vi "glavni_program.vi"() -> ()   [LabVIEW 2019]
uses:
  vrste_kafe.ctl
  stanja.ctl
  <vilib>/DAQmx/read.llb/DAQmx Read (Analog 1D DBL 1Chan NSamp).vi
  <vilib>/DAQmx/read.llb/DAQmx Read (Analog DBL 1Chan 1Samp).vi
  <vilib>/DAQmx/miscellaneous.llb/DAQmx Fill In Error Info.vi
  <vilib>/DAQmx/create/channels.llb/DAQmx Create Channel (AI-Voltage-Basic).vi
  <vilib>/DAQmx/configure/timing.llb/DAQmx Timing (Sample Clock).vi
panel:
  out "temperatura":dbl
  out "zapremina":dbl
  out "vreme kafe":i32
  in  "izbor kraci/duzi":bool
  in  "duzi espresso":bool
  out "vreme zagrevanja[ms]":u32
  out "start time":u32
  in  "stop":bool
  in  "Broj kafa":T1
  in  "Izbor kafe":T2
  in  "Ukljuci":bool
  out "L2":bool
  in  "Otkloni gresku":bool
  in  "Pravi kafu":bool
  in  "Zagrej vodu":bool
  in  "Ubaci kapsulu":bool
  out "Lampice":T3
  in  "Dopuni":bool
  out "L1":bool
  # "kraći espresso"
  # "duži espresso"
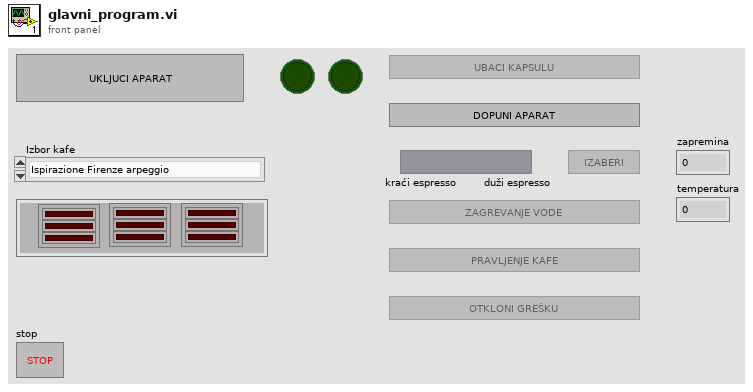
[diagram p1: front panel]
types:
  T1 = cluster{"Vrsta1":dbl, "Vrsta 2":dbl, "Vrsta 3":dbl}
  T2 = typedef "vrste_kafe.ctl" = enum16{"Ispirazione Firenze arpeggio", "Barista Corto", "Ispirazione Napoli"}
  T3 = cluster{"3 lampice":cluster{"led3coffee1":bool, "led2coffee1":bool, "led1coffee1":bool}, "3 lampice 2":cluster{"led3coffee1":bool, "led2coffee1":bool, "led1coffee1":bool}, "3 lampice 3":cluster{"led3coffee1":bool, "led2coffee1":bool, "led1coffee1":bool}}
  T4 = enum16{"open", "replace", "create", "open or create", "replace or create", "replace or create with confirmation"}
  T5 = typedef "stanja.ctl" = enum16{"Inicijalizacija", "Cekanje", "Ubaci kapsulu", "Izbor slike kapsule", "Zapremina vode", "Zagrevanje vode", "Pravljenje kafe", "Zavrsetak"}
  T6 = enum8{"Enabled", "Disabled", "Disabled and Grayed Out"}
  T7 = cluster{"Vrsta1":dbl, "Vrsta2":dbl, "Vrsta3":dbl}
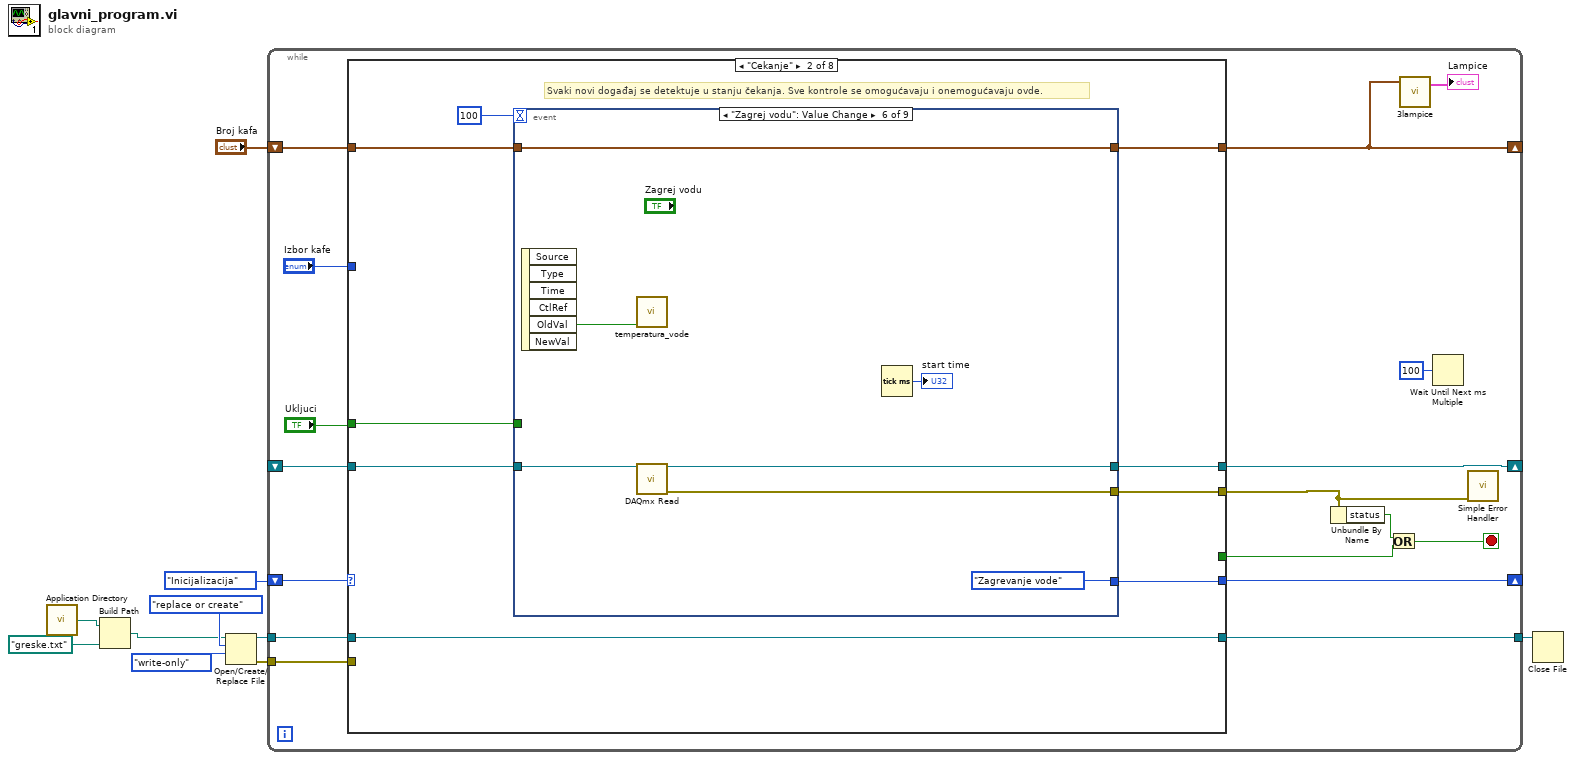
[diagram p0: block diagram]
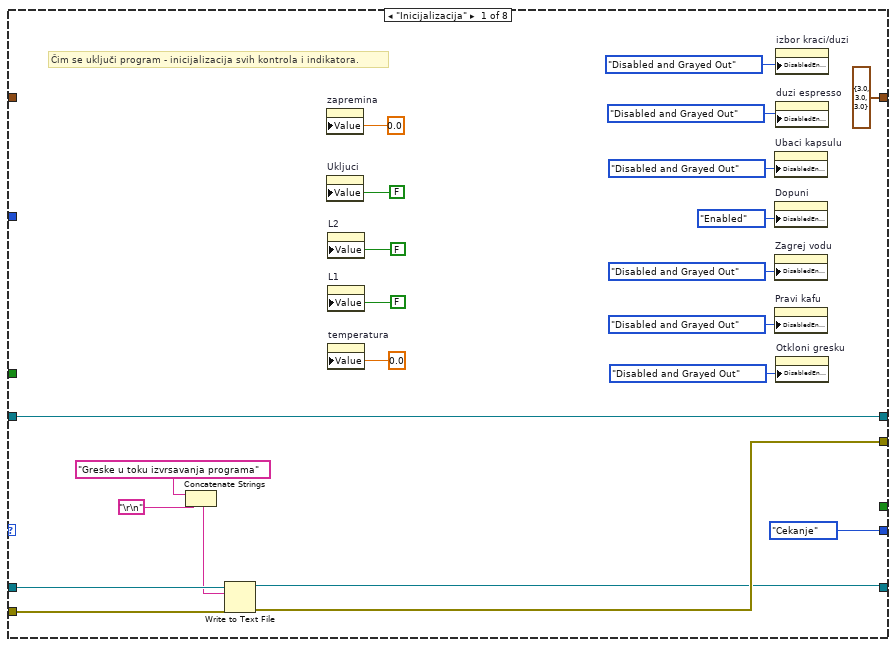
[diagram p2: hidden frame]
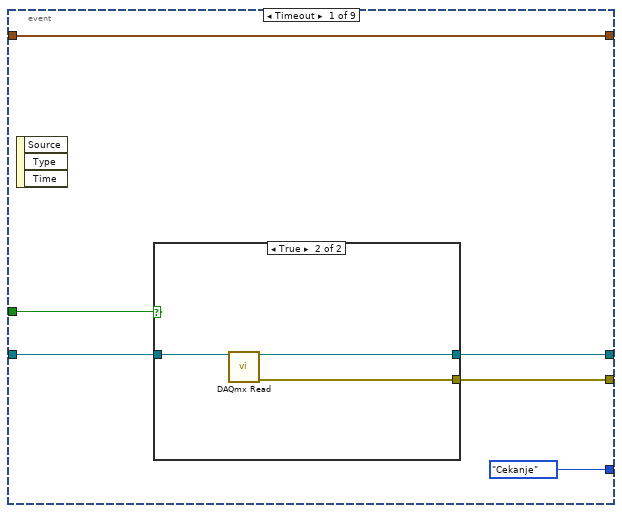
[diagram p3: hidden frame]
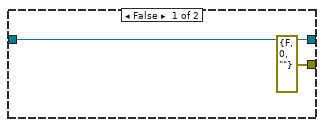
[diagram p4: hidden frame]
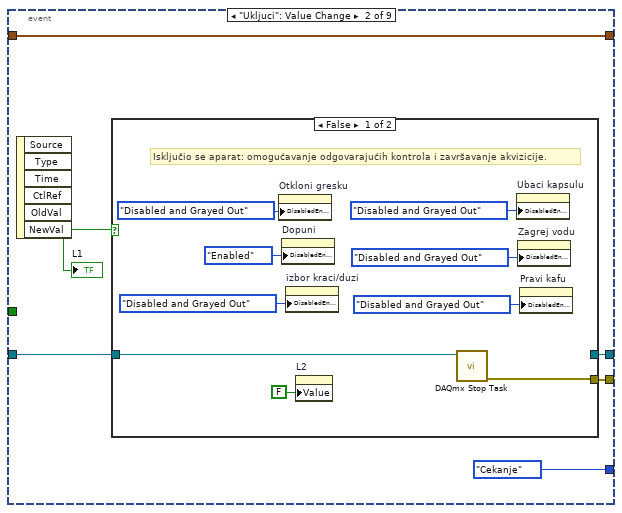
[diagram p5: hidden frame]
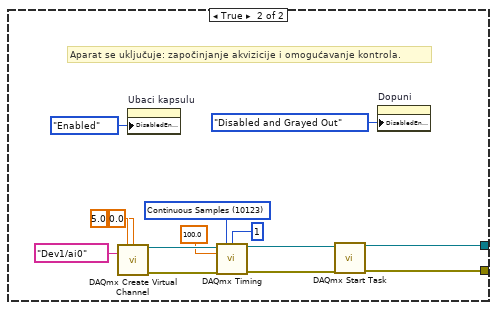
[diagram p6: hidden frame]
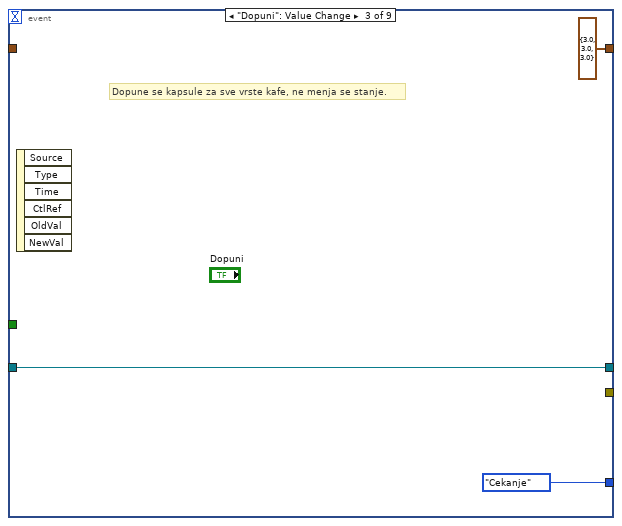
[diagram p7: hidden frame]
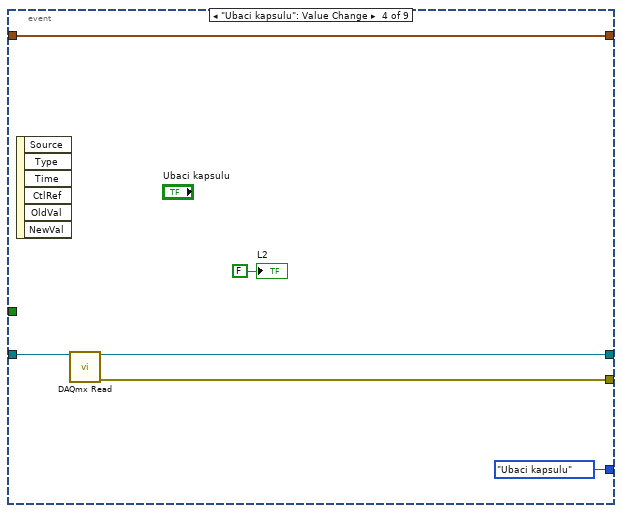
[diagram p8: hidden frame]
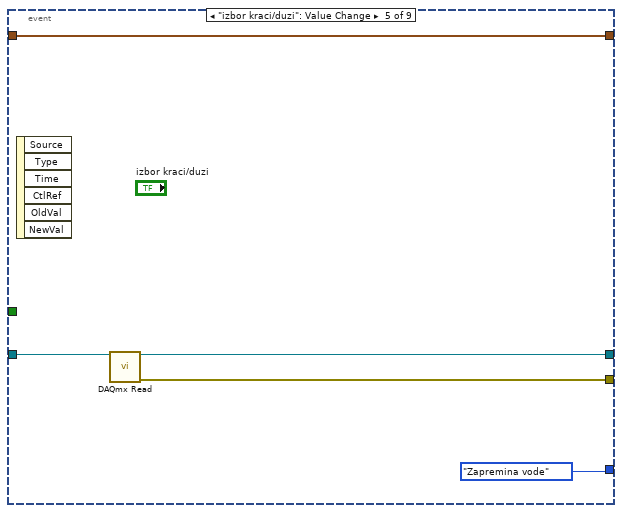
[diagram p9: hidden frame]
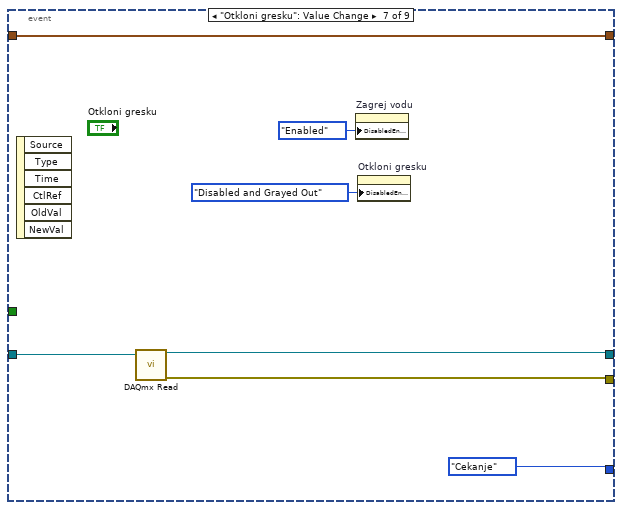
[diagram p10: hidden frame]
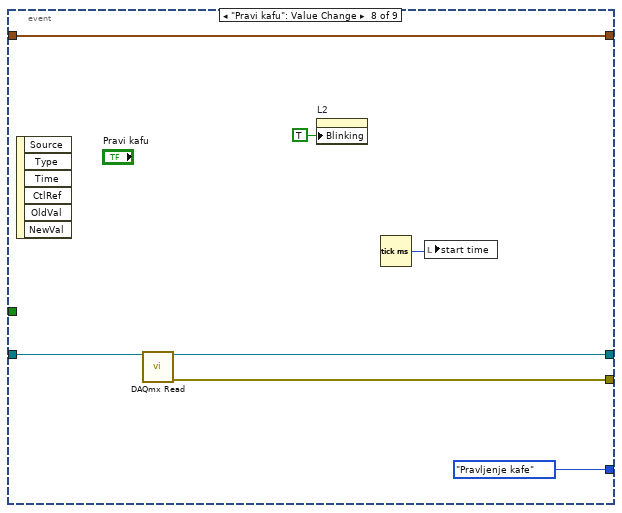
[diagram p11: hidden frame]
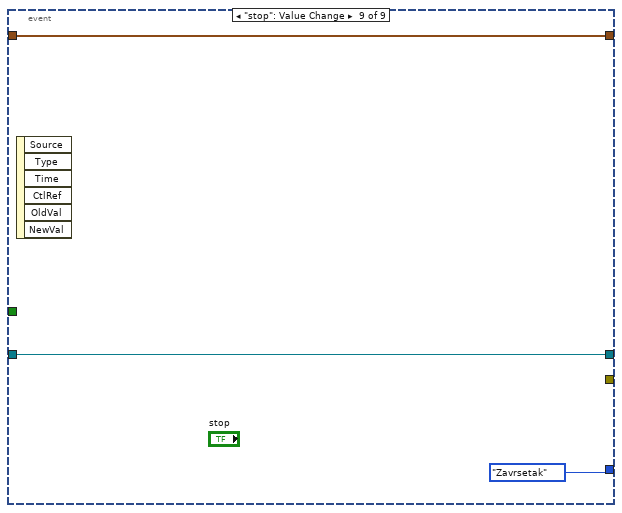
[diagram p12: hidden frame]
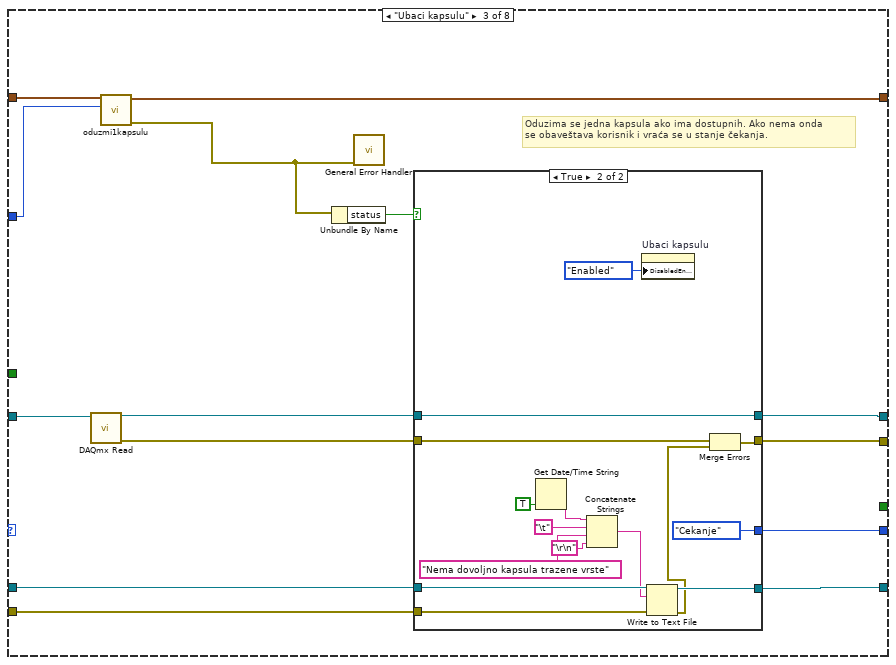
[diagram p13: hidden frame]
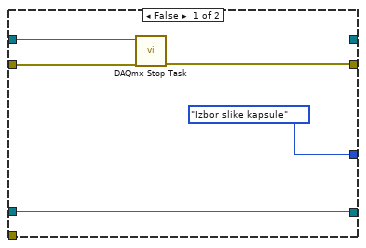
[diagram p14: hidden frame]
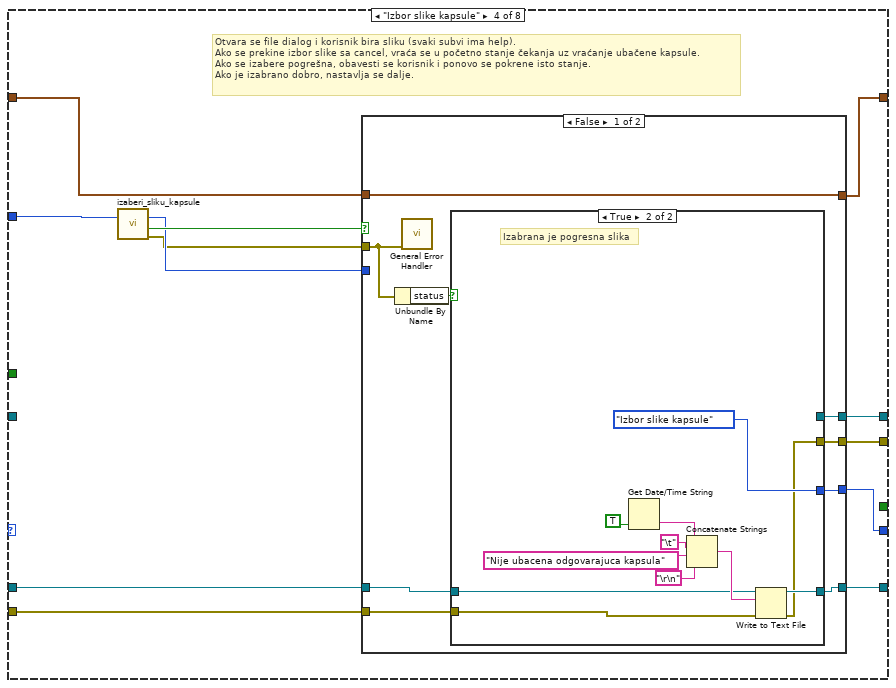
[diagram p15: hidden frame]
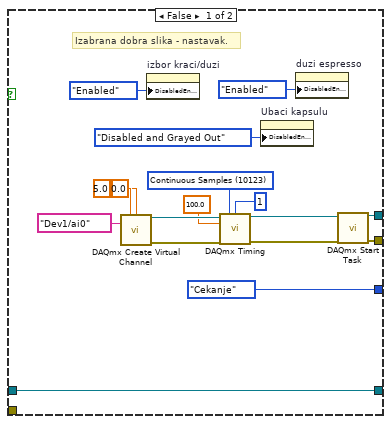
[diagram p16: hidden frame]
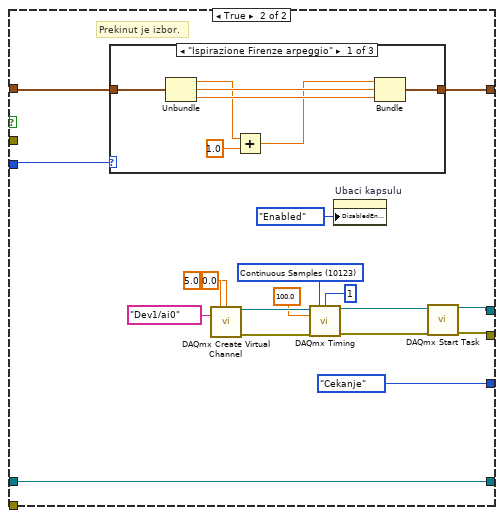
[diagram p17: hidden frame]
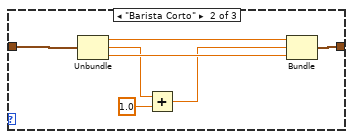
[diagram p18: hidden frame]
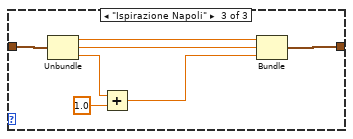
[diagram p19: hidden frame]
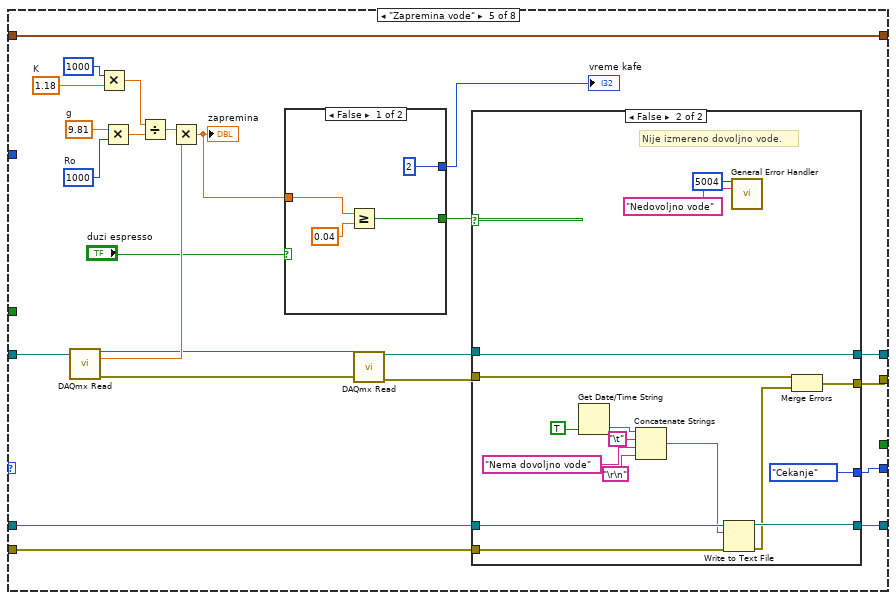
[diagram p20: hidden frame]
diagram:
  n1 = call <vilib>:"Application Directory.vi"() -> ("Application Directory"=w2:path)
  n2 = Build Path(base path=w2, name or relative path=path "greske.txt" ("file path (use dialog)")) -> (appended path=w1:path)
  n3 = Open/Create/Replace File(file path (use dialog)=w1, operation (0:open)=T4."replace or create", access (0:read/write)=enum16{"read/write", "read-only", "write-only"}."write-only") -> (refnum out=w6:refnum<file>, error out=w5:errorcluster)  [unwired: 3 in, 1 out]
  n4 = while {
    shift-right: [w26] -> _
    shift-left: stanja."Inicijalizacija" ("Stanja sistema") -> [w27]
    shift-right: [w25] -> _
    shift-left: _ -> [w22]
    shift-right: [w17] -> _
    shift-left: "Broj kafa" -> [w16]
    tunnel: w6 -> [w13]
    tunnel: w5 -> [w12]
    tunnel: [w11] -> w4
    stop <- w24 stop-if-true
    n5 = case shown="\"Cekanje\"" w27 {
      tunnel: [stanja."Cekanje" ("Stanja sistema") w57 w145 w176 w267 w318 w366 stanja."Inicijalizacija" ("Stanja sistema")] -> w26
      tunnel: [w48 w56 w142 w175 w263 w320 w373 _] -> w25
      tunnel: [w32 w55 w140 w174 w262 w313 w372 w384] -> w21
      tunnel: w22 -> [w48 w54 w147 _ w272 w321 w374 w398]
      tunnel: [T1 {"Vrsta1"=3.0, "Vrsta 2"=3.0, "Vrsta 3"=3.0} ("Broj kafa") w51 w149 w179 w281 w323 w375 T1 {"Vrsta1"=0.0, "Vrsta 2"=0.0, "Vrsta 3"=0.0} ("Broj kafa")] -> w17
      tunnel: "Ukljuci" -> [_ w53 _ _ _ _ _ w399]
      tunnel: [_ _ _ _ _ _ _ TRUE] -> w18
      tunnel: w16 -> [_ w52 w150 w177 w281 w323 w375 _]
      tunnel: "Izbor kafe" -> [_ _ w148 w180 _ _ _ _]
      tunnel: w13 -> [w34 w50 w139 w171 w266 w317 w371 w383]
      tunnel: w12 -> [w33 _ w138 w173 w264 _ _ _]
      tunnel: [w31 w50 w137 w172 w265 w316 w371 w383] -> w11
      frame "Inicijalizacija" {
        # "Čim se uključi program - inicijalizacija svih kontrola i indikatora."
        n6 = Concatenate Strings("Greske u toku izvrsavanja programa" ("string"), "\r\n") -> (w29:string)
        n7 = Write to Text File(file (use dialog)=w34, text=w29, error in=w33) -> (refnum out=w31:refnum<file>, error out=w32:errorcluster)  [unwired: 1 in, 1 out]
        n8 = property on="zapremina" class="DigNum (strict)"("Value"=0.0 ("zapremina")) -> ()  [unwired: 2 in, 2 out]
        n9 = property on="Ukljuci" class="Bool (strict)"("Value"=FALSE ("Ukljuci")) -> ()  [unwired: 2 in, 2 out]
        n10 = property on="L2" class="Bool (strict)"("Value"=FALSE ("L2")) -> ()  [unwired: 2 in, 2 out]
        n11 = property on="L1" class="Bool (strict)"("Value"=FALSE ("L1")) -> ()  [unwired: 2 in, 2 out]
        n12 = property on="temperatura" class="DigNum (strict)"("Value"=0.0 ("Temperature")) -> ()  [unwired: 2 in, 2 out]
        n13 = property on="Ubaci kapsulu" class="Bool"("DisabledEnum"=T6."Disabled and Grayed Out" ("Disabled")) -> ()  [unwired: 2 in, 2 out]
        n14 = property on="Dopuni" class="Bool"("DisabledEnum"=T6."Enabled" ("Disabled")) -> ()  [unwired: 2 in, 2 out]
        n15 = property on="Zagrej vodu" class="Bool"("DisabledEnum"=T6."Disabled and Grayed Out" ("Disabled")) -> ()  [unwired: 2 in, 2 out]
        n16 = property on="Pravi kafu" class="Bool"("DisabledEnum"=T6."Disabled and Grayed Out" ("Disabled")) -> ()  [unwired: 2 in, 2 out]
        n17 = property on="izbor kraci/duzi" class="Bool"("DisabledEnum"=T6."Disabled and Grayed Out" ("Disabled")) -> ()  [unwired: 2 in, 2 out]
        n18 = property on="duzi espresso" class="Bool (strict)"("DisabledEnum"=T6."Disabled and Grayed Out" ("Disabled")) -> ()  [unwired: 2 in, 2 out]
        n19 = property on="Otkloni gresku" class="Bool"("DisabledEnum"=T6."Disabled and Grayed Out" ("Disabled")) -> ()  [unwired: 2 in, 2 out]
      }
      frame "Cekanje" {
        # "Svaki novi događaj se detektuje u stanju čekanja. Sve kontrole se omogućavaju i onemogućavaju ovde."
        n20 = event shown="[5] \"Zagrej vodu\": Value Change" {
          selector: _ -> [_ _ _ _ _ _ _ _ _]
          dyn-events: _ -> [_ _ _ _ _ _ _ _ _]
          timeout: 100 -> [_ _ _ _ _ _ _ _ _]
          tunnel: [stanja."Cekanje" ("Stanja sistema") stanja."Cekanje" ("Stanja sistema") stanja."Cekanje" ("Stanja sistema") stanja."Ubaci kapsulu" ("Stanja sistema") stanja."Zapremina vode" ("Stanja sistema") stanja."Zagrevanje vode" ("Stanja sistema") stanja."Cekanje" ("Stanja sistema") stanja."Pravljenje kafe" ("Stanja sistema") stanja."Zavrsetak" ("Stanja sistema")] -> w57
          tunnel: [w62 w74 w99 w106 w111 w117 w122 w132 w135] -> w56
          tunnel: [w61 w73 _ w105 w110 w116 w120 w131 _] -> w55
          tunnel: w54 -> [w63 w72 w99 w107 w112 w118 w123 w133 w135]
          tunnel: w53 -> [w60 _ _ _ _ _ _ _ _]
          tunnel: w52 -> [w59 w70 _ w103 w108 w119 w121 w129 w134]
          tunnel: [w59 w70 T7 {"Vrsta1"=3.0, "Vrsta2"=3.0, "Vrsta3"=3.0} ("Broj kafa izlaz") w103 w108 w119 w121 w129 w134] -> w51
          event Timeout {
            n21 = event-data() -> ()  [unwired: 1 in, 3 out]
            n22 = case shown="True" w60 {
              tunnel: w63 -> [w66 w69]
              tunnel: [w66 w68] -> w62
              tunnel: [errorcluster {"status"=FALSE, "code"=0, "source"=""} ("error out") w67] -> w61
              frame False {
              }
              frame True {
                n23 = call-poly <vilib>:"DAQmx Read.vi"("task/channels in"=w69) -> ("task out"=w68:refnum<k21>, "error out"=w67:errorcluster)  [unwired: 12 in, 1 out]
              }
            }
          }
          event "Ukljuci": Value Change {
            n24 = event-data() -> ("NewVal"=w71:bool)  [unwired: 1 in, 5 out]
            "L1" <- w71
            n25 = case shown="False" w71 {
              tunnel: [_ w87] -> w74
              tunnel: [w83 w86] -> w73
              tunnel: w72 -> [w84 _]
              frame False {
                # "Isključio se aparat: omogućavanje odgovarajućih kontrola i završavanje akvizicije."
                n26 = property on="Otkloni gresku" class="Bool"("DisabledEnum"=T6."Disabled and Grayed Out" ("Disabled")) -> ()  [unwired: 2 in, 2 out]
                n27 = property on="Dopuni" class="Bool"("DisabledEnum"=T6."Enabled" ("Disabled")) -> ()  [unwired: 2 in, 2 out]
                n28 = property on="izbor kraci/duzi" class="Bool"("DisabledEnum"=T6."Disabled and Grayed Out" ("Disabled")) -> ()  [unwired: 2 in, 2 out]
                n29 = property on="L2" class="Bool (strict)"("Value"=FALSE ("L2")) -> ()  [unwired: 2 in, 2 out]
                n30 = call <vilib>:"DAQmx Stop Task.vi"("task/channels in"=w84) -> ("error out"=w83:errorcluster)  [unwired: 13 in, 1 out]
                n31 = property on="Ubaci kapsulu" class="Bool"("DisabledEnum"=T6."Disabled and Grayed Out" ("Disabled")) -> ()  [unwired: 2 in, 2 out]
                n32 = property on="Zagrej vodu" class="Bool"("DisabledEnum"=T6."Disabled and Grayed Out" ("Disabled")) -> ()  [unwired: 2 in, 2 out]
                n33 = property on="Pravi kafu" class="Bool"("DisabledEnum"=T6."Disabled and Grayed Out" ("Disabled")) -> ()  [unwired: 2 in, 2 out]
              }
              frame True {
                w91 = 10123 items=["Finite Samples"=10178, "Continuous Samples"=10123, "Hardware Timed Single Point"=12522] ("sample mode")
                # "Aparat se uključuje: započinjanje akvizicije i omogućavanje kontrola."
                n34 = call-poly <vilib>:"DAQmx Create Virtual Channel.vi"("maximum value"=5.0, "minimum value"=0.0, "physical channels"=tag "Dev1/ai0") -> ("task out"=w95:refnum<k21>, "error out"=w96:errorcluster)  [unwired: 11 in]
                n35 = property on="Ubaci kapsulu" class="Bool"("DisabledEnum"=T6."Enabled" ("Disabled")) -> ()  [unwired: 2 in, 2 out]
                n36 = call-poly <vilib>:"DAQmx Timing.vi"("task/channels in"=w95, "sample mode"=w91, "samples per channel"=1, "rate"=100.0, "error in"=w96) -> ("task out"=w97:refnum<k21>, "error out"=w98:errorcluster)  [unwired: 9 in]
                n37 = call <vilib>:"DAQmx Start Task.vi"("task/channels in"=w97, "error in"=w98) -> ("task out"=w87:refnum<k21>, "error out"=w86:errorcluster)  [unwired: 12 in]
                n38 = property on="Dopuni" class="Bool"("DisabledEnum"=T6."Disabled and Grayed Out" ("Disabled")) -> ()  [unwired: 2 in, 2 out]
              }
            }
          }
          event "Dopuni": Value Change {
            # "Dopune se kapsule za sve vrste kafe, ne menja se stanje."
            n39 = event-data() -> ()  [unwired: 1 in, 6 out]
          }
          event "Ubaci kapsulu": Value Change {
            n40 = event-data() -> ()  [unwired: 1 in, 6 out]
            n41 = call-poly <vilib>:"DAQmx Read.vi"("task/channels in"=w107) -> ("task out"=w106:refnum<k21>, "error out"=w105:errorcluster)  [unwired: 12 in, 1 out]
            "L2" <- FALSE ("L2")
          }
          event "izbor kraci/duzi": Value Change {
            n42 = event-data() -> ()  [unwired: 1 in, 6 out]
            n43 = call-poly <vilib>:"DAQmx Read.vi"("task/channels in"=w112) -> ("task out"=w111:refnum<k21>, "error out"=w110:errorcluster)  [unwired: 12 in, 1 out]
          }
          event "Zagrej vodu": Value Change {
            n44 = event-data() -> ("OldVal"=w113:bool)  [unwired: 1 in, 5 out]
            n45 = call "temperatura_vode.vi"("Heating"=w113) -> ()  [unwired: 10 in, 1 out]
            n46 = call-poly <vilib>:"DAQmx Read.vi"("task/channels in"=w118) -> ("task out"=w117:refnum<k21>, "error out"=w116:errorcluster)  [unwired: 12 in, 1 out]
            n47 = Tick Count (ms)() -> (millisecond timer value=→"start time":u32)
          }
          event "Otkloni gresku": Value Change {
            n48 = event-data() -> ()  [unwired: 1 in, 6 out]
            n49 = call-poly <vilib>:"DAQmx Read.vi"("task/channels in"=w123) -> ("task out"=w122:refnum<k21>, "error out"=w120:errorcluster)  [unwired: 12 in, 1 out]
            n50 = property on="Zagrej vodu" class="Bool"("DisabledEnum"=T6."Enabled" ("Disabled")) -> ()  [unwired: 2 in, 2 out]
            n51 = property on="Otkloni gresku" class="Bool"("DisabledEnum"=T6."Disabled and Grayed Out" ("Disabled")) -> ()  [unwired: 2 in, 2 out]
          }
          event "Pravi kafu": Value Change {
            n52 = event-data() -> ()  [unwired: 1 in, 6 out]
            n53 = call-poly <vilib>:"DAQmx Read.vi"("task/channels in"=w133) -> ("task out"=w132:refnum<k21>, "error out"=w131:errorcluster)  [unwired: 12 in, 1 out]
            n54 = property on="L2" class="Bool (strict)"("Blinking"=TRUE) -> ()  [unwired: 2 in, 2 out]
            n55 = Tick Count (ms)() -> (millisecond timer value=w128:u32)
            n56 = local write "start time"(w128) -> ()
          }
          event "stop": Value Change {
            n57 = event-data() -> ()  [unwired: 1 in, 6 out]
          }
        }
      }
      frame "Ubaci kapsulu" {
        # "Oduzima se jedna kapsula ako ima dostupnih. Ako nema onda\nse obaveštava korisnik i vraća se u stanje čekanja."
        n58 = call-poly <vilib>:"DAQmx Read.vi"("task/channels in"=w147) -> ("task out"=w143:refnum<k21>, "error out"=w141:errorcluster)  [unwired: 12 in, 1 out]
        n59 = call "oduzmi1kapsulu.vi"("Izbor kafe"=w148, "Broj kafa ulaz"=w150) -> ("error out"=w144:errorcluster, "Broj kafa izlaz"=w149:T7)  [unwired: 8 in]
        n60 = Unbundle By Name(w144) -> ("status"=w146:bool)
        n61 = call <vilib>:"General Error Handler.vi"("error in (no error)"=w144) -> ()  [unwired: 10 in, 5 out]
        n62 = case shown="True" w146 {
          tunnel: [stanja."Izbor slike kapsule" ("Stanja sistema") stanja."Cekanje" ("Stanja sistema")] -> w145
          tunnel: w143 -> [w154 w168]
          tunnel: [_ w168] -> w142
          tunnel: w141 -> [w153 w164]
          tunnel: [w152 w163] -> w140
          tunnel: w139 -> [w151 w167]
          tunnel: w138 -> [_ w166]
          tunnel: [w151 w165] -> w137
          frame False {
            n63 = call <vilib>:"DAQmx Stop Task.vi"("task/channels in"=w154, "error in"=w153) -> ("error out"=w152:errorcluster)  [unwired: 12 in, 1 out]
          }
          frame True {
            n64 = Get Date/Time String(want seconds? (F)=TRUE) -> (time string=w161:string)  [unwired: 2 in, 1 out]
            n65 = Concatenate Strings(w161, "\t", "Nema dovoljno kapsula trazene vrste" ("string"), "\r\n") -> (w160:string)
            n66 = property on="Ubaci kapsulu" class="Bool"("DisabledEnum"=T6."Enabled" ("Disabled")) -> ()  [unwired: 2 in, 2 out]
            n67 = Write to Text File(file (use dialog)=w167, text=w160, error in=w166) -> (refnum out=w165:refnum<file>, error out=w162:errorcluster)  [unwired: 1 in, 1 out]
            n68 = Merge Errors(w164, w162) -> (w163:errorcluster)
          }
        }
      }
      frame "Izbor slike kapsule" {
        # "Otvara se file dialog i korisnik bira sliku (svaki subvi ima help). \nAko se prekine izbor slike sa cancel, vraća se u početno stanje čekanja uz vraćanje ubačene kapsule. \nAko se izabere pogrešna, obavesti se korisnik i ponovo se pokrene isto stanje.\nAko je izabrano dobro, nastavlja se dalje."
        n69 = call "izaberi_sliku_kapsule.vi"("Izbor kafe ulaz"=w180) -> ("error out"=w178:errorcluster, "prekinut"=w181:bool)  [unwired: 8 in, 1 out]
        n70 = case shown="False" w181 {
          tunnel: w180 -> [_ w220]
          tunnel: [w190 w236] -> w179
          tunnel: w178 -> [w189 _]
          tunnel: [w187 stanja."Cekanje" ("Stanja sistema")] -> w176
          tunnel: w177 -> [w190 w233]
          tunnel: [w186 w222] -> w175
          tunnel: [w185 w221] -> w174
          tunnel: w173 -> [w184 _]
          tunnel: [w183 w219] -> w172
          tunnel: w171 -> [w182 w219]
          frame False {
            n71 = Unbundle By Name(w189) -> ("status"=w188:bool)
            n72 = call <vilib>:"General Error Handler.vi"("error in (no error)"=w189) -> ()  [unwired: 10 in, 5 out]
            n73 = case shown="True" w188 {
              tunnel: [stanja."Cekanje" ("Stanja sistema") stanja."Izbor slike kapsule" ("Stanja sistema")] -> w187
              tunnel: [w194 _] -> w186
              tunnel: [w193 w210] -> w185
              tunnel: w184 -> [_ w212]
              tunnel: [w191 w211] -> w183
              tunnel: w182 -> [w191 w208]
              frame False {
                w197 = 10123 items=["Finite Samples"=10178, "Continuous Samples"=10123, "Hardware Timed Single Point"=12522] ("sample mode")
                # "Izabrana dobra slika - nastavak."
                n74 = call-poly <vilib>:"DAQmx Create Virtual Channel.vi"("maximum value"=5.0, "minimum value"=0.0, "physical channels"=tag "Dev1/ai0") -> ("task out"=w201:refnum<k21>, "error out"=w202:errorcluster)  [unwired: 11 in]
                n75 = property on="izbor kraci/duzi" class="Bool"("DisabledEnum"=T6."Enabled" ("Disabled")) -> ()  [unwired: 2 in, 2 out]
                n76 = call-poly <vilib>:"DAQmx Timing.vi"("task/channels in"=w201, "sample mode"=w197, "samples per channel"=1, "rate"=100.0, "error in"=w202) -> ("task out"=w203:refnum<k21>, "error out"=w204:errorcluster)  [unwired: 9 in]
                n77 = property on="Ubaci kapsulu" class="Bool"("DisabledEnum"=T6."Disabled and Grayed Out" ("Disabled")) -> ()  [unwired: 2 in, 2 out]
                n78 = property on="duzi espresso" class="Bool (strict)"("DisabledEnum"=T6."Enabled" ("Disabled")) -> ()  [unwired: 2 in, 2 out]
                n79 = call <vilib>:"DAQmx Start Task.vi"("task/channels in"=w203, "error in"=w204) -> ("task out"=w194:refnum<k21>, "error out"=w193:errorcluster)  [unwired: 12 in]
              }
              frame True {
                # "Izabrana je pogresna slika"
                n80 = Get Date/Time String(want seconds? (F)=TRUE) -> (time string=w216:string)  [unwired: 2 in, 1 out]
                n81 = Concatenate Strings(w216, "\t", "Nije ubacena odgovarajuca kapsula" ("string"), "\r\n") -> (w209:string)
                n82 = Write to Text File(file (use dialog)=w208, text=w209, error in=w212) -> (refnum out=w211:refnum<file>, error out=w210:errorcluster)  [unwired: 1 in, 1 out]
              }
            }
          }
          frame True {
            w225 = 10123 items=["Finite Samples"=10178, "Continuous Samples"=10123, "Hardware Timed Single Point"=12522] ("sample mode")
            # "Prekinut je izbor."
            n83 = case shown="\"Ispirazione Firenze arpeggio\"" w220 {
              tunnel: [w237 w244 w251] -> w236
              tunnel: w233 -> [w239 w246 w253]
              frame "Ispirazione Firenze arpeggio" {
                n84 = Unbundle(w239) -> ("Vrsta1"=w238:dbl, "Vrsta 2"=w242:dbl, "Vrsta 3"=w243:dbl)
                n85 = Add(x=w238, y=1.0) -> (x+y=w240:dbl)
                n86 = Bundle(w240, "Vrsta 2"=w242, "Vrsta 3"=w243) -> (w237:cluster{dbl, "Vrsta 2":dbl, "Vrsta 3":dbl})  [unwired: 1 in]
              }
              frame "Barista Corto" {
                n87 = Unbundle(w246) -> ("Vrsta1"=w247:dbl, "Vrsta 2"=w245:dbl, "Vrsta 3"=w250:dbl)
                n88 = Add(x=w245, y=1.0) -> (x+y=w248:dbl)
                n89 = Bundle("Vrsta1"=w247, w248, "Vrsta 3"=w250) -> (w244:cluster{"Vrsta1":dbl, dbl, "Vrsta 3":dbl})  [unwired: 1 in]
              }
              frame "Ispirazione Napoli" {
                n90 = Unbundle(w253) -> ("Vrsta1"=w254:dbl, "Vrsta 2"=w257:dbl, "Vrsta 3"=w252:dbl)
                n91 = Add(x=w252, y=1.0) -> (x+y=w255:dbl)
                n92 = Bundle("Vrsta1"=w254, "Vrsta 2"=w257, w255) -> (w251:cluster{"Vrsta1":dbl, "Vrsta 2":dbl, dbl})  [unwired: 1 in]
              }
            }
            n93 = call-poly <vilib>:"DAQmx Create Virtual Channel.vi"("maximum value"=5.0, "minimum value"=0.0, "physical channels"=tag "Dev1/ai0") -> ("task out"=w229:refnum<k21>, "error out"=w230:errorcluster)  [unwired: 11 in]
            n94 = call-poly <vilib>:"DAQmx Timing.vi"("task/channels in"=w229, "sample mode"=w225, "samples per channel"=1, "rate"=100.0, "error in"=w230) -> ("task out"=w231:refnum<k21>, "error out"=w232:errorcluster)  [unwired: 9 in]
            n95 = property on="Ubaci kapsulu" class="Bool"("DisabledEnum"=T6."Enabled" ("Disabled")) -> ()  [unwired: 2 in, 2 out]
            n96 = call <vilib>:"DAQmx Start Task.vi"("task/channels in"=w231, "error in"=w232) -> ("task out"=w222:refnum<k21>, "error out"=w221:errorcluster)  [unwired: 12 in]
          }
        }
      }
      frame "Zapremina vode" {
        w277 = 1000  # Ro
        w276 = 9.81  # g
        w275 = 1.18  # K
        n97 = call-poly <vilib>:"DAQmx Read.vi"("task/channels in"=w272) -> ("task out"=w261:refnum<k21>, "data"=w280:dbl, "error out"=w260:errorcluster)  [unwired: 12 in]
        n98 = Multiply(x=1000, y=w275) -> (x*y=w279:dbl)
        n99 = Multiply(x=w276, y=w277) -> (x*y=w278:dbl)
        n100 = Divide(x=w279, y=w278) -> (x/y=w273:dbl)
        n101 = Multiply(x=w273, y=w280) -> (x*y=w271:dbl)
        "zapremina" <- w271
        n102 = case shown="False" "duzi espresso" {
          tunnel: w271 -> [w307 w311]
          tunnel: [w305 w310] -> w269
          tunnel: [2 4] -> w268
          frame False {
            n103 = Greater Or Equal?(x=w307, y=0.04) -> (x >= y?=w305:bool)
          }
          frame True {
            n104 = Greater Or Equal?(x=w311, y=0.11) -> (x >= y?=w310:bool)
          }
        }
        "vreme kafe" <- w268
        n105 = call-poly <vilib>:"DAQmx Read.vi"("task/channels in"=w261, "error in"=w260) -> ("task out"=w259:refnum<k21>, "error out"=w258:errorcluster)  [unwired: 11 in, 1 out]
        n106 = case shown="False" w269 {
          tunnel: [stanja."Cekanje" ("Stanja sistema") stanja."Cekanje" ("Stanja sistema")] -> w267
          tunnel: w266 -> [w284 w300]
          tunnel: [w284 w301] -> w265
          tunnel: w264 -> [_ w299]
          tunnel: w259 -> [w283 w298]
          tunnel: [w283 w298] -> w263
          tunnel: w258 -> [w282 w296]
          tunnel: [w282 w297] -> w262
          frame True {
            # "Sve prošlo okej."
            n107 = property on="duzi espresso" class="Bool (strict)"("DisabledEnum"=T6."Disabled and Grayed Out" ("Disabled")) -> ()  [unwired: 2 in, 2 out]
            n108 = property on="izbor kraci/duzi" class="Bool"("DisabledEnum"=T6."Disabled and Grayed Out" ("Disabled")) -> ()  [unwired: 2 in, 2 out]
            n109 = property on="Zagrej vodu" class="Bool"("DisabledEnum"=T6."Enabled" ("Disabled")) -> ()  [unwired: 2 in, 2 out]
          }
          frame False {
            # "Nije izmereno dovoljno vode."
            n110 = Get Date/Time String(want seconds? (F)=TRUE) -> (time string=w292:string)  [unwired: 2 in, 1 out]
            n111 = Concatenate Strings(w292, "\t", "Nema dovoljno vode" ("string"), "\r\n") -> (w294:string)
            n112 = Write to Text File(file (use dialog)=w300, text=w294, error in=w299) -> (refnum out=w301:refnum<file>, error out=w295:errorcluster)  [unwired: 1 in, 1 out]
            n113 = call <vilib>:"General Error Handler.vi"("[error code] (0)"=5004, "[error source] (\" \")"="Nedovoljno vode" ("[error source] (\" \")")) -> ()  [unwired: 9 in, 5 out]
            n114 = Merge Errors(w296, w295) -> (w297:errorcluster)
          }
        }
      }
      frame "Zagrevanje vode" {
        w319 = TRUE
        n115 = call-poly <vilib>:"DAQmx Read.vi"("task/channels in"=w321) -> ("task out"=w320:refnum<k21>, "error out"=w315:errorcluster)  [unwired: 12 in, 1 out]
        n116 = call "temperatura_vode.vi"("Heating"=w319) -> ("Temperature"=w322:dbl)  [unwired: 10 in]
        n117 = case shown="True" w319 {
          tunnel: w322 -> [_ w332]
          tunnel: [stanja."Zagrevanje vode" ("Stanja sistema") w329] -> w318
          tunnel: w317 -> [w324 w328]
          tunnel: [w324 w327] -> w316
          tunnel: [_ w326] -> w314
          frame False {
          }
          frame True {
            # "ovaj case je samo da bi se cekao rezultat\nmerenja temperature pre odredjivanja vremena"
            n118 = local read "start time"() -> (w331:u32)
            n119 = Tick Count (ms)() -> (millisecond timer value=w330:u32)
            n120 = Subtract(x=w330, y=w331) -> (x-y=w335:u32)
            "vreme zagrevanja[ms]" <- w335
            n121 = Greater Or Equal?(x=w335, y=u32 10000) -> (x >= y?=w333:bool)
            n122 = Greater Or Equal?(x=w332, y=85.0) -> (x >= y?=w336:bool)
            n123 = case shown="False" w336 {
              tunnel: w333 -> [w342 _]
              tunnel: [w341 stanja."Cekanje" ("Stanja sistema")] -> w329
              tunnel: w328 -> [w340 w359]
              tunnel: [w339 w359] -> w327
              tunnel: [w338 _] -> w326
              frame False {
                n124 = case shown="True" w342 {
                  tunnel: [stanja."Cekanje" ("Stanja sistema") stanja."Zagrevanje vode" ("Stanja sistema")] -> w341
                  tunnel: w340 -> [w346 w357]
                  tunnel: [w345 w357] -> w339
                  tunnel: [w343 _] -> w338
                  frame True {
                    n125 = Get Date/Time String(want seconds? (F)=TRUE) -> (time string=w350:string)  [unwired: 2 in, 1 out]
                    n126 = Concatenate Strings(w350, "\t", "Problem sa grejacem" ("string"), "\r\n") -> (w344:string)
                    n127 = Write to Text File(file (use dialog)=w346, text=w344) -> (refnum out=w345:refnum<file>, error out=w343:errorcluster)  [unwired: 2 in, 1 out]
                    n128 = property on="Otkloni gresku" class="Bool"("DisabledEnum"=T6."Enabled" ("Disabled")) -> ()  [unwired: 2 in, 2 out]
                    n129 = call <vilib>:"Simple Error Handler.vi"("error code (no error:0)"=5005, "error source (\" \")"="Problem sa aparatom" ("error source (\" \")")) -> ()  [unwired: 3 in, 5 out]
                    n130 = property on="Zagrej vodu" class="Bool"("DisabledEnum"=T6."Disabled and Grayed Out" ("Disabled")) -> ()  [unwired: 2 in, 2 out]
                  }
                  frame False {
                  }
                }
              }
              frame True {
                n131 = property on="Pravi kafu" class="Bool"("DisabledEnum"=T6."Enabled" ("Disabled")) -> ()  [unwired: 2 in, 2 out]
                n132 = property on="Zagrej vodu" class="Bool"("DisabledEnum"=T6."Disabled and Grayed Out" ("Disabled")) -> ()  [unwired: 2 in, 2 out]
              }
            }
            "temperatura" <- w332
          }
        }
        n133 = Merge Errors(w315, w314) -> (w313:errorcluster)
      }
      frame "Pravljenje kafe" {
        n134 = call-poly <vilib>:"DAQmx Read.vi"("task/channels in"=w374) -> ("task out"=w373:refnum<k21>, "error out"=w372:errorcluster)  [unwired: 12 in, 1 out]
        n135 = local read "start time"() -> (w369:u32)
        n136 = local read "vreme kafe"() -> (w365:i32)
        n137 = Tick Count (ms)() -> (millisecond timer value=w370:u32)
        n138 = Subtract(x=w370, y=w369) -> (x-y=w368:u32)
        n139 = Multiply(x=1000, y=w365) -> (x*y=w363:i32)
        n140 = Greater Or Equal?(x=w368, y=w363) -> (x >= y?=w367:bool)
        n141 = case shown="False" w367 {
          tunnel: [stanja."Pravljenje kafe" ("Stanja sistema") stanja."Cekanje" ("Stanja sistema")] -> w366
          frame False {
          }
          frame True {
            n142 = property on="L2" class="Bool (strict)"("Blinking"=FALSE, "Value"=TRUE ("L2")) -> (error out=w379:errorcluster)  [unwired: 2 in, 1 out]
            n143 = property on="Pravi kafu" class="Bool"("DisabledEnum"=T6."Disabled and Grayed Out" ("Disabled")) -> ()  [unwired: 2 in, 2 out]
            n144 = property on="Ubaci kapsulu" class="Bool"(error in=w379, "DisabledEnum"=T6."Enabled" ("Disabled")) -> ()  [unwired: 1 in, 2 out]
          }
        }
      }
      frame "Zavrsetak" {
        # "Pre isključivanja programa, sve kontrole se vraćaju u osnovno stanje (kao na početku).\nAko nije završena akvizicija završava se ovde."
        # "posle ovoga kraj"
        # "poslato bilo koje stanje"
        n145 = case shown="False" w399 {
          tunnel: w398 -> [w400 w402]
          tunnel: [w400 w401] -> w385
          frame False {
          }
          frame True {
            # "Ukljucen je aparat - znaci da nije zavrsena\nakvizicija pa se ovde zatvara."
            n146 = call <vilib>:"DAQmx Stop Task.vi"("task/channels in"=w402) -> ("task out"=w401:refnum<k21>)  [unwired: 13 in, 1 out]
          }
        }
        n147 = property on="L2" class="Bool (strict)"("Value"=FALSE ("L2"), "Blinking"=FALSE) -> ()  [unwired: 2 in, 2 out]
        n148 = property on="L1" class="Bool (strict)"("Value"=FALSE ("L1")) -> ()  [unwired: 2 in, 2 out]
        n149 = property on="Ukljuci" class="Bool (strict)"("Value"=FALSE ("Ukljuci")) -> ()  [unwired: 2 in, 2 out]
        n150 = call <vilib>:"DAQmx Clear Task.vi"("task in"=w385) -> ("error out"=w384:errorcluster)  [unwired: 14 in]
        n151 = property on="Ubaci kapsulu" class="Bool"("DisabledEnum"=T6."Disabled and Grayed Out" ("Disabled")) -> ()  [unwired: 2 in, 2 out]
        n152 = property on="Dopuni" class="Bool"("DisabledEnum"=T6."Enabled" ("Disabled")) -> ()  [unwired: 2 in, 2 out]
        n153 = property on="Zagrej vodu" class="Bool"("DisabledEnum"=T6."Disabled and Grayed Out" ("Disabled")) -> ()  [unwired: 2 in, 2 out]
        n154 = property on="Otkloni gresku" class="Bool"("DisabledEnum"=T6."Disabled and Grayed Out" ("Disabled")) -> ()  [unwired: 2 in, 2 out]
        n155 = property on="Pravi kafu" class="Bool"("DisabledEnum"=T6."Disabled and Grayed Out" ("Disabled")) -> ()  [unwired: 2 in, 2 out]
      }
    }
    n156 = Unbundle By Name(w21) -> ("status"=w23:bool)
    n157 = Or(x=w23, y=w18) -> (x .or. y?=w24:bool)
    n158 = call "3lampice.vi"("Cluster"=w17) -> ("Lampice"=→"Lampice":T3)  [unwired: 4 in]
    n159 = Wait Until Next ms Multiple(millisecond multiple=u32 100) -> ()  [unwired: 1 out]
    n160 = call <vilib>:"Simple Error Handler.vi"("error in (no error)"=w21) -> ()  [unwired: 4 in, 5 out]
  }
  n161 = Close File(refnum=w4) -> ()  [unwired: 1 in, 2 out]
